vi "simple_FFT.vi"(1 "element":dbl[](array[numeric])) -> (0 "X":cdb[](array[numeric]))   [LabVIEW 2013, in "varilib.lvlib"]
doc: "Simple script based FFT. Uses Cooley-Tukey radix-2 Decimation-In-Time algorithm. Will work only for data sets of length N = 2^M, where M is integer."
uses:
  varilib.lvlib
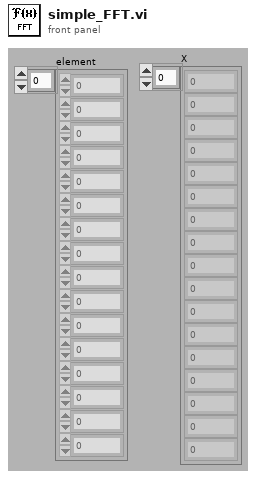
[diagram p1: front panel]
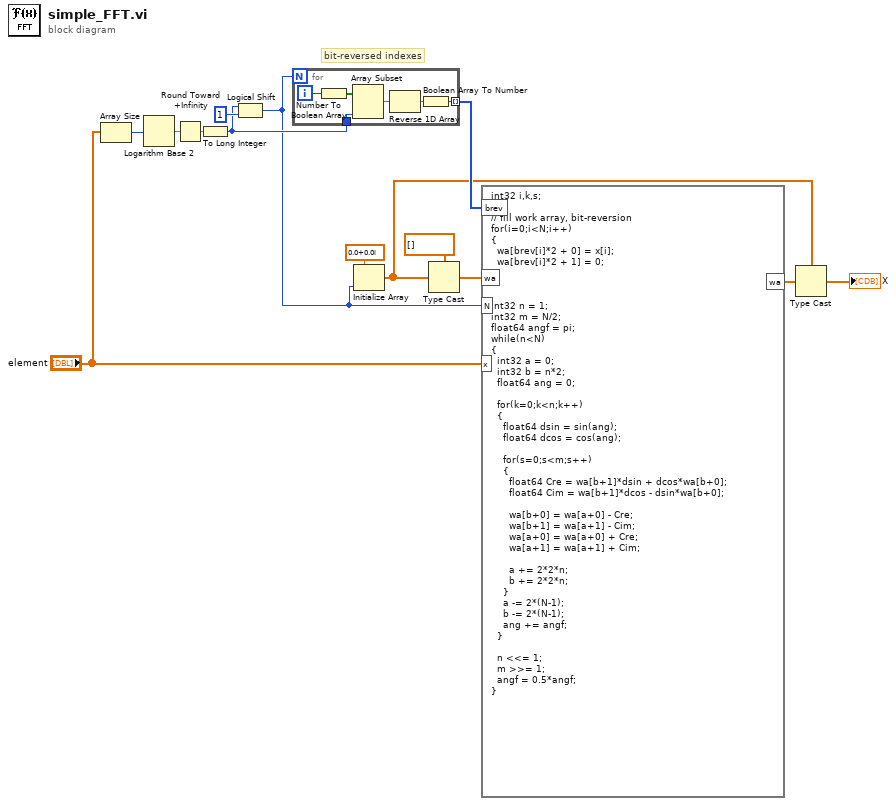
[diagram p0: block diagram]
diagram:
  # "bit-reversed indexes"
  n1 = Array Size(array="element") -> (size(s)=w3:i32)
  n2 = Logarithm Base 2(1:w3) -> (0:w9:dbl)
  n3 = Round Toward +Infinity(x=w9) -> (ceil(x): smallest int >= x=w8:dbl)
  n4 = To Long Integer(number=w8) -> (32bit integer=w6:i32)
  n5 = Logical Shift(y=w6, x=u32 1) -> (x << y=w4:u32)
  n6 = for {
    N: w4 -> [_]
    tunnel: w6 -> [w19]
    tunnel: [w16] -> w13 mode=indexing
    i -> [w15]
    n7 = Number To Boolean Array(number=w15) -> (Boolean array=w20:bool[])
    n8 = Array Subset(array=w20, length=w19) -> (w18:bool[])  [unwired: 1 in]
    n9 = Reverse 1D Array(array=w18) -> (reversed array=w17:bool[])
    n10 = Boolean Array To Number(Boolean array=w17) -> (number=w16:u32)
  }
  n11 = Initialize Array(cdb 0.0+0.0i ("element"), w4) -> (w10:cdb[])
  n12 = Type Cast(type=dbl[] [], x=w10) -> (*(type *) &x=w12:dbl[])
  n13 = formula code="int32 i,k,s;\n\n// fill work array, bit-reversion\nfor(i=0;i<N;i++)\n{\n  wa[brev[i]*2 + 0] = x[i];\n  wa[brev[i]*2 + 1] = 0;\n}\n\n\nint32 n = 1;\nint32 m = N/2;\nfloat64 angf = pi;\nwhile(n<N)\n{\n  int32 a = 0;\n  int32 b = n*2;\n  float64 ang = 0;\n\n  for(k=0;k<n;k++)\n  {\n    float64 dsin = sin(ang);\n    float64 dcos = cos(ang);\n\n    for(s=0;s<m;s++)\n    {\n      float64 Cre = wa[b+1]*dsin + dcos*wa[b+0];\n      float64 Cim = wa[b+1]*dcos - dsin*wa[b+0];\n      \n      wa[b+0] = wa[a+0] - Cre;\n      wa[b+1] = wa[a+1] - Cim;\n      wa[a+0] = wa[a+0] + Cre;\n      wa[a+1] = wa[a+1] + Cim;\n      \n      a += 2*2*n;\n      b += 2*2*n;\n    }\n    a -= 2*(N-1);\n    b -= 2*(N-1);\n    ang += angf;\n  }\n\n  n <<= 1;\n  m >>= 1;\n  angf = 0.5*angf;\n}"("x"="element", "N"=w4, "wa"=w12, "brev"=w13) -> ("wa"=w5:dbl[])
  n14 = Type Cast(type=w10, x=w5) -> (*(type *) &x=→"X":cdb[])
